vi "Servo Call.vi"(0 "Travel (Degree)":dbl=100.0, 1 "Speed d/s":dbl=10.0, 2 "Mode":i32(ring)=10178 items=["Finite Samples"=10178, "Continuous Samples"=10123, "Hardware Timed Single Point"=12522], 3 "error in":errorcluster, 4 "Servo On Bit":bool) -> (9 "error out":errorcluster)   [LabVIEW 2015]
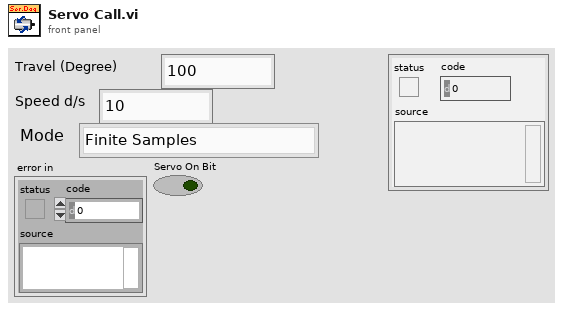
[diagram p1: front panel]
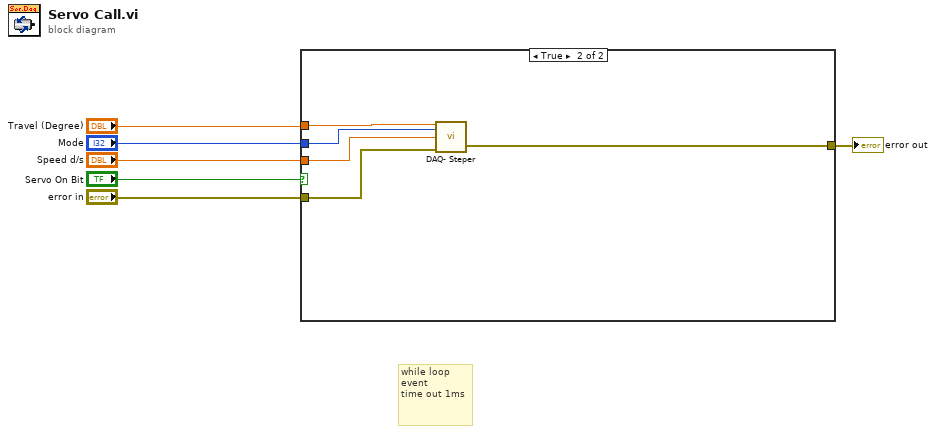
[diagram p0: block diagram]
diagram:
  # "while loop  \nevent\ntime out 1ms"
  n1 = case shown="True" "Servo On Bit" {
    tunnel: [w7 w12] -> w6
    tunnel: "Mode" -> [_ w11]
    tunnel: "Travel (Degree)" -> [_ w10]
    tunnel: "Speed d/s" -> [_ w9]
    tunnel: "error in" -> [w7 w8]
    frame False {
    }
    frame True {
      n2 = call "DAQ- Steper.vi"("Travel (Degree)"=w10, "Mode"=w11, "Speed d/s"=w9, "error in"=w8) -> ("error out"=w12:errorcluster)  [unwired: 10 in, 1 out]
    }
  }
  "error out" <- w6
